vi "Configure SubAddress.vi"(5 "Word Count\\Mode Code":T4, 7 "SubAddress":T3, 8 "Parameter Prefix":string, 11 "Command Type":T2) -> (3 "SubAddress Configuration":T1={"Command Type"=enum."Transmit", "SubAddress"=enum."1", "Word Count\\Mode Code"=enum."1", "Initial Data"=[], "Data Fields"=[]} {"Data Fields"."Base Word" format="%04d"; "Initial Data" format="%04x"})   [LabVIEW 2020, in "BCI-1553 RealTime API Examples.lvlib"]
uses:
  BCI-1553 RealTime API Examples.lvlib
  src/RealTime/Frames & Messages/TypeDefs/Command Word Count.ctl
  src/RealTime/Frames & Messages/TypeDefs/Command SubAddress.ctl
  src/RealTime/Frames & Messages/TypeDefs/Command Type.ctl
  src/RealTime/Remote Terminal/TypeDefs/RT Command Config.ctl
  src/RealTime/Frames & Messages/TypeDefs/Simplified Parameter Data Table.ctl
  src/RealTime/Frames & Messages/TypeDefs/Scaling Information.ctl
  src/RealTime/BCI-1553 API.lvlib
  src/RealTime/Remote Terminal/Remote Terminal.lvclass
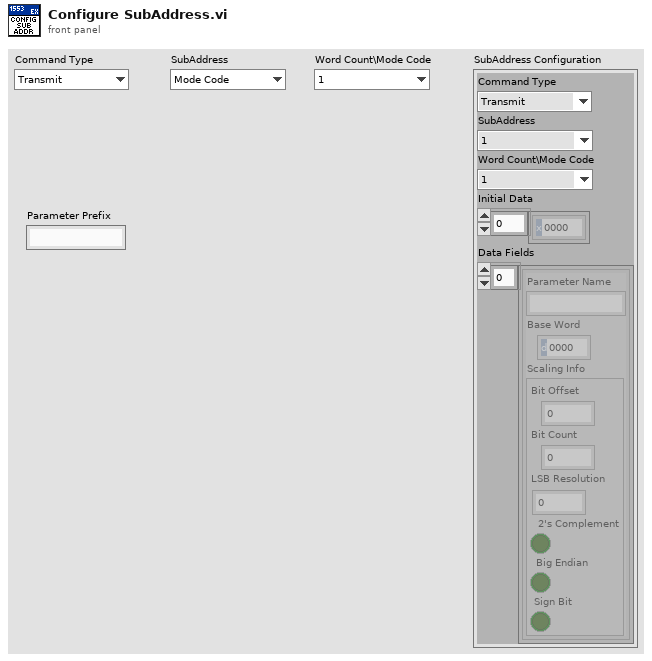
[diagram p1: front panel]
types:
  T1 = typedef "BCI-1553 API.lvlib/Remote Terminal.lvclass/RT Command Config.ctl" = cluster{"Command Type":T2, "SubAddress":T3, "Word Count\\Mode Code":T4, "Initial Data":u16[], "Data Fields":T5[]}
  T2 = typedef "BCI-1553 API.lvlib/Command Type.ctl" = enum16{"Transmit", "Receive"}
  T3 = typedef "BCI-1553 API.lvlib/Command SubAddress.ctl" = enum16{"Mode Code", "1", "2", "3", "4", "5", "6", "7", "8", "9", "10", "11", "12", "13", "14", "15", "16", "17", "18", "19", "20", "21", "22", "23", "24", "25", "26", "27", "28", "29", "30"}
  T4 = typedef "BCI-1553 API.lvlib/Command Word Count.ctl" = enum16{"1", "2", "3", "4", "5", "6", "7", "8", "9", "10", "11", "12", "13", "14", "15", "16", "17", "18", "19", "20", "21", "22", "23", "24", "25", "26", "27", "28", "29", "30", "31", "32"}
  T5 = typedef "BCI-1553 API.lvlib/Simplified Parameter Data Table.ctl" = cluster{"Parameter Name":string, "Base Word":u16, "Scaling Info":T6}
  T6 = typedef "BCI-1553 API.lvlib/Scaling Information.ctl" = cluster{"Bit Offset":i32, "Bit Count":i32, "LSB Resolution":dbl, "2's Complement":bool, "Big Endian":bool, "Sign Bit":bool}
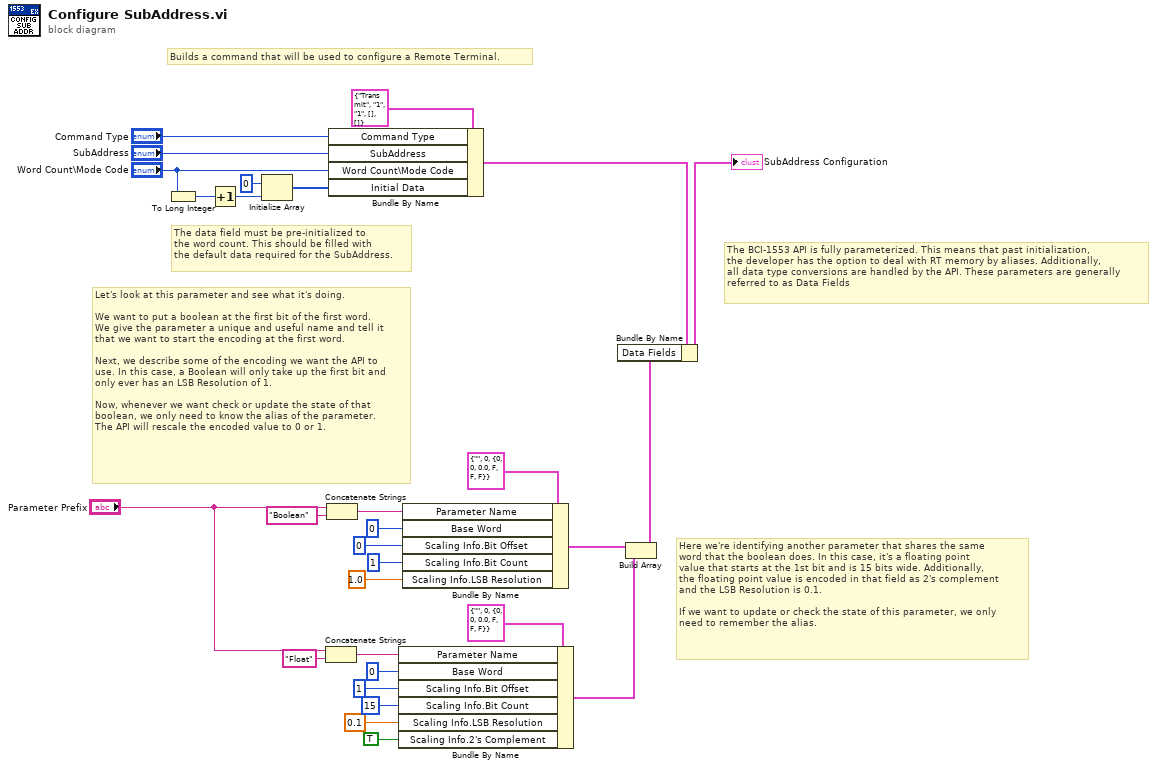
[diagram p0: block diagram]
diagram:
  # "The BCI-1553 API is fully parameterized. This means that past initialization,\nthe developer has the option to deal with RT memory by aliases. Additionally,\nall data type conversions are handled by the API. These parameters are generally\nreferred to as Data Fields"
  # "Here we're identifying another parameter that shares the same\nword that the boolean does. In this case, it's a floating point\nvalue that starts at the 1st bit and is 15 bits wide. Additionally,\nthe floating point value is encoded in that field as 2's complement\nand the LSB Resolution is 0.1.\n\nIf we want to update or check the state of this parameter, we only\nneed to remember the alias."
  # "Let's look at this parameter and see what it's doing.\n\nWe want to put a boolean at the first bit of the first word.\nWe give the parameter a unique and useful name and tell it\nthat we want to start the encoding at the first word.\n\nNext, we describe some of the encoding we want the API to\nuse. In this case, a Boolean will only take up the first bit and\nonly ever has an LSB Resolution of 1.\n\nNow, whenever we want check or update the state of that\nboolean, we only need to know the alias of the parameter.\nThe API will rescale the encoded value to 0 or 1."
  # "Builds a command that will be used to configure a Remote Terminal."
  # "The data field must be pre-initialized to\nthe word count. This should be filled with\nthe default data required for the SubAddress."
  n1 = To Long Integer(number="Word Count\\Mode Code") -> (32bit integer=w28:i32)
  n2 = Increment(x=w28) -> (x+1=w26:i32)
  n3 = Initialize Array(u16 0 ("element"), w26) -> (w7:u16[])
  n4 = Concatenate Strings("Parameter Prefix", "Float" ("string")) -> (w13:string)
  n5 = Concatenate Strings("Parameter Prefix", "Boolean" ("string")) -> (w22:string)
  n6 = Bundle By Name(cluster=T1 {"Command Type"=enum."Transmit", "SubAddress"=enum."1", "Word Count\\Mode Code"=enum."1", "Initial Data"=[], "Data Fields"=[]} ("CMD Configuration"), "Command Type"="Command Type", "SubAddress"="SubAddress", "Word Count\\Mode Code"="Word Count\\Mode Code", "Initial Data"=w7) -> (w29:T1)
  n7 = Bundle By Name(cluster=T5 {"Parameter Name"="", "Base Word"=0, "Scaling Info"={"Bit Offset"=0, "Bit Count"=0, "LSB Resolution"=0.0, "2's Complement"=FALSE, "Big Endian"=FALSE, "Sign Bit"=FALSE}} ("Parameter Data Table"), "Parameter Name"=w13, "Base Word"=u16 0, "Scaling Info.Bit Offset"=1, "Scaling Info.Bit Count"=15, "Scaling Info.LSB Resolution"=0.1, "Scaling Info.2's Complement"=TRUE) -> (w12:T5)
  n8 = Bundle By Name(cluster=T5 {"Parameter Name"="", "Base Word"=0, "Scaling Info"={"Bit Offset"=0, "Bit Count"=0, "LSB Resolution"=0.0, "2's Complement"=FALSE, "Big Endian"=FALSE, "Sign Bit"=FALSE}} ("Parameter Data Table"), "Parameter Name"=w22, "Base Word"=u16 0, "Scaling Info.Bit Offset"=0, "Scaling Info.Bit Count"=1, "Scaling Info.LSB Resolution"=1.0) -> (w11:T5)
  n9 = Build Array(w11, w12) -> (w10:T5[])
  n10 = Bundle By Name(cluster=w29, "Data Fields"=w10) -> (→"SubAddress Configuration":T1)
